vi "Configure Deskew Sensitivity.vi"(7 "Vertical Sensitivity (1.0 V)":dbl=1.0, 8 "error in (no error)":errorcluster, 9 "Deskew Time (0)":dbl, 10 "Channel (0: Channel 1)":i32(ring) items=["Channel 1", "Channel 2", "Channel 3", "Channel 4"], 11 "VISA resource name":refnum<visa-resource-name>) -> (0 "error out":errorcluster, 3 "VISA resource name out":refnum<visa-resource-name>)   [LabVIEW 2016, in "Tektronix DPO MSO 2000 4000 Series.lvlib"]
doc: "Configures the deskew time and vertical sensitivity of the oscilloscope for the channel you specified."
uses:
  Tektronix DPO MSO 2000 4000 Series.lvlib
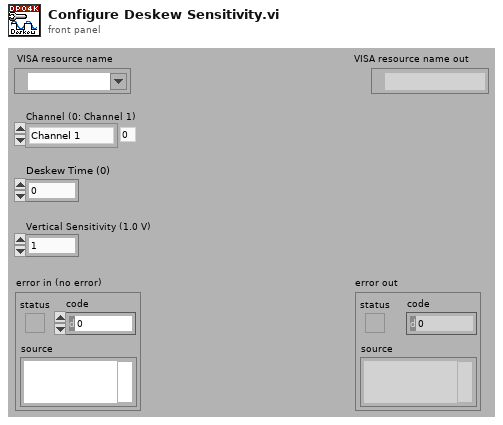
[diagram p1: front panel]
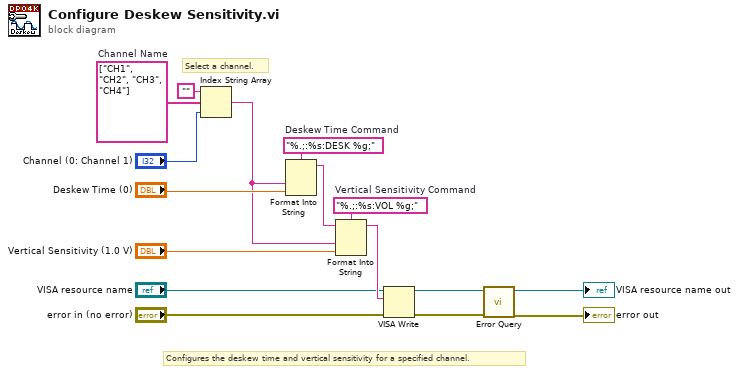
[diagram p0: block diagram]
diagram:
  w4 = string[] ["CH1", "CH2", "CH3", "CH4"]  # Channel Name
  w13 = "%.;:%s:VOL %g;"  # Vertical Sensitivity Command
  w16 = "%.;:%s:DESK %g;"  # Deskew Time Command
  # "Select a channel."
  # "Configures the deskew time and vertical sensitivity for a specified channel."
  n1 = Index String Array(1:"Channel (0: Channel 1)", 2:w4, 3:"") -> (0:w1:string)
  n2 = Format Into String(format string=w16, w1, "Deskew Time (0)") -> (resulting string=w14:string)  [unwired: 2 in, 1 out]
  n3 = Format Into String(format string=w13, initial string=w14, w1, "Vertical Sensitivity (1.0 V)") -> (resulting string=w11:string)  [unwired: 1 in, 1 out]
  n4 = VISA Write(VISA resource name="VISA resource name", write buffer=w11, error in (no error)="error in (no error)") -> (VISA resource name out=w8:refnum<visa-resource-name>, error out=w7:errorcluster)  [unwired: 1 out]
  n5 = call "Error Query.vi"("error in (no error)"=w7, "VISA resource name"=w8) -> ("error out"=→"error out":errorcluster, "VISA resource name out"=→"VISA resource name out":refnum<visa-resource-name>)  [unwired: 6 in, 2 out]
